vi "LJLogM build log data string.vi"(1 "Data":dbl[][](array[numeric]) format="%.2f") -> (0 "Output data":string)   [LabVIEW 2026]
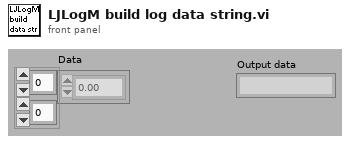
[diagram p1: front panel]
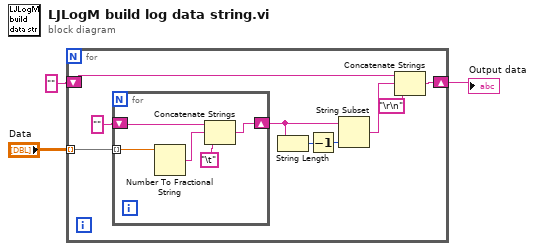
[diagram p0: block diagram]
diagram:
  n1 = for {
    tunnel: "Data" -> [w12] mode=indexing
    shift-right: [w8] -> w1
    shift-left: "" -> [w7]
    n2 = for {
      shift-right: [w14] -> w9
      shift-left: "" -> [w15]
      tunnel: w12 -> [w17] mode=indexing
      n3 = Number To Fractional String(number=w17) -> (F-format string=w16:string)  [unwired: 3 in]
      n4 = Concatenate Strings(w15, w16, "\t") -> (w14:string)
    }
    n5 = String Length(string=w9) -> (length=w10:i32)
    n6 = Decrement(x=w10) -> (x-1=w11:i32)
    n7 = String Subset(string=w9, length (rest)=w11) -> (substring=w6:string)  [unwired: 1 in]
    n8 = Concatenate Strings(w7, w6, "\r\n") -> (w8:string)
  }
  "Output data" <- w1
